vi "Initiate Trigger System.vi"(8 "error in (no error)":errorcluster, 10 "Trigger State (0: Single)":u16(ring) items=["Single", "Continuous", "Idle"], 11 "VISA resource name":refnum<visa-resource-name>) -> (0 "error out":errorcluster, 3 "VISA resource name out":refnum<visa-resource-name>)   [LabVIEW 2017, in "HH PLI Series.lvlib"]
doc: "Initiates the trigger system to single, continuous or idle state."
uses:
  HH PLI Series.lvlib
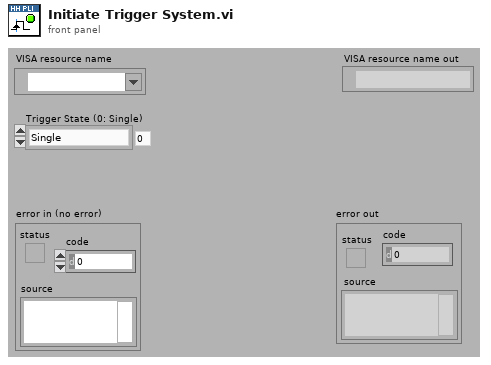
[diagram p1: front panel]
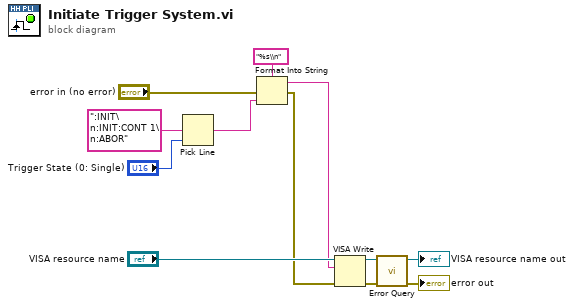
[diagram p0: block diagram]
diagram:
  n1 = Pick Line(multi-line string=":INIT\n:INIT:CONT 1\n:ABOR" ("command"), line index="Trigger State (0: Single)") -> (output string=w1:string)  [unwired: 1 in]
  n2 = Format Into String(format string="%s\\n", error in="error in (no error)", w1) -> (resulting string=w7:string, error out=w5:errorcluster)  [unwired: 1 in]
  n3 = VISA Write(VISA resource name="VISA resource name", write buffer=w7, error in (no error)=w5) -> (VISA resource name out=w10:refnum<visa-resource-name>, error out=w11:errorcluster)  [unwired: 1 out]
  n4 = call "Error Query.vi"("error in (no error)"=w11, "VISA resource name"=w10) -> ("error out"=→"error out":errorcluster, "VISA resource name out"=→"VISA resource name out":refnum<visa-resource-name>)  [unwired: 6 in, 2 out]
